vi "Initialize Transfer Group.vi"(5 "FIFO Options":T1, 6 "Transfer Group Status":refnum<class "Transfer Group Status.lvclass">, 7 "id":i32, 8 "error in (no error)":errorcluster, 9 "force inline? (F)":bool, 10 "Transfer Group Buffers":refnum<class "Buffers.lvclass">, 11 "Transfer Group Configuration":T2={"name"="", "direction"=enum."Tx", "cycle timing"={"priority"=0, "decimation"=1, "offset"=0}, "thread"=-1, "settings"=[], "Transfers"=[]} {"Transfers"."channels"."string offset" format="%d bytes"}) -> (0 "error out":errorcluster, 3 "Transfer Group out":refnum<class "Transfer Group.lvclass">)   [LabVIEW 2017, in "DSF Core.lvlib" / "Transfer Group.lvclass"]
uses:
  Transfer Group.lvclass
  Typedefs/DSF Engine Transfer Group Configuration.ctl
  Typedefs/DSF Direction.ctl
  Typedefs/DSF Timing Info.ctl
  Typedefs/DSF Settings Info.ctl
  Typedefs/DSF Engine Transfer Configuration.ctl
  Typedefs/DSF Byte Order.ctl
  Typedefs/DSF Engine Channel Configuration.ctl
  Typedefs/DSF Data Type.ctl
  Buffer/Buffers.lvclass
  Typedefs/DSF FIFO Options.ctl
  Transfer Group Status/Transfer Group Status.lvclass
  Configuration/Required Buffer Size (Transfer).vi
  Transfer/Transfer.lvclass
  DSF Core.lvlib
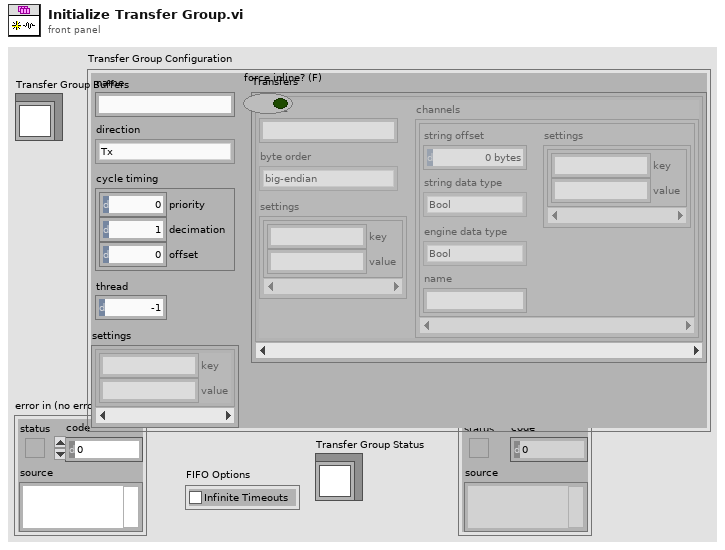
[diagram p1: front panel]
types:
  T1 = typedef "DSF Core.lvlib/DSF FIFO Options.ctl" = cluster{"Infinite Timeouts":bool}
  T2 = typedef "DSF Core.lvlib/DSF Engine Transfer Group Configuration.ctl" = cluster{"name":string, "direction":T3, "cycle timing":T4, "thread":i32, "settings":T5, "Transfers":T6[]}
  T3 = typedef "DSF Core.lvlib/DSF Direction.ctl" = enum8{"Tx", "Rx"}
  T4 = typedef "DSF Core.lvlib/DSF Timing Info.ctl" = cluster{"priority":u64, "decimation":u64, "offset":u64}
  T5 = typedef "DSF Core.lvlib/DSF Settings Info.ctl" = cluster{"key":string, "value":string}[]
  T6 = typedef "DSF Core.lvlib/DSF Engine Transfer Configuration.ctl" = cluster{"name":string, "byte order":T7, "settings":T5, "channels":T8[]}
  T7 = typedef "DSF Core.lvlib/DSF Byte Order.ctl" = enum8{"big-endian", "little-endian"}
  T8 = typedef "DSF Core.lvlib/DSF Engine Channel Configuration.ctl" = cluster{"string offset":u64, "string data type":T9, "engine data type":T9, "name":string, "settings":T5}
  T9 = typedef "DSF Core.lvlib/DSF Data Type.ctl" = enum8{"Bool", "SGL", "DBL", "I8", "I16", "I32", "I64", "U8", "U16", "U32", "U64"}
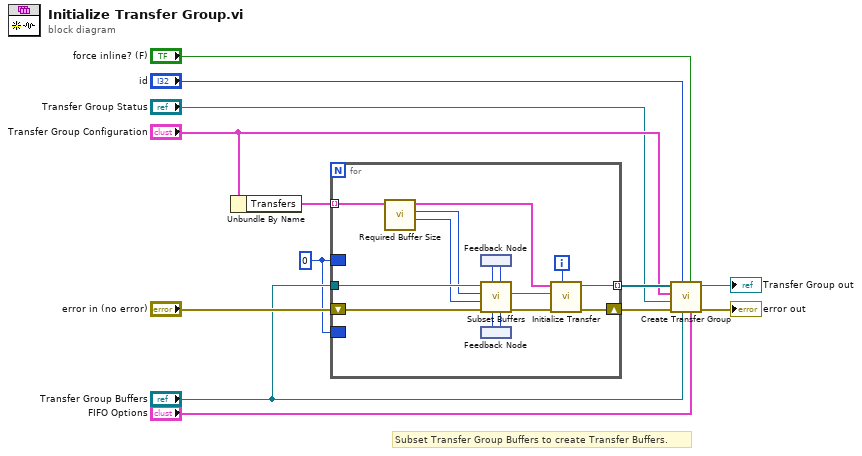
[diagram p0: block diagram]
diagram:
  w6 = u64 0 ("inline buffer size")
  # "Subset Transfer Group Buffers to create Transfer Buffers."
  n1 = Unbundle By Name("Transfer Group Configuration") -> ("Transfers"=w11:T6[])
  n2 = for {
    tunnel: w11 -> [w25] mode=indexing
    tunnel: [w28] -> w9 mode=indexing
    shift-right: [w27] -> w10
    shift-left: "error in (no error)" -> [w23]
    border: w6 -> [_]
    border: w6 -> [_]
    tunnel: "Transfer Group Buffers" -> [w22]
    i -> [w26]
    n3 = call-poly "Required Buffer Size.vi"("Transfer Configuration in"=w25) -> ("total engine buffer size"=w14:u64, "total string buffer size"=w15:u64, "Transfer Configuration out"=w24:T6)  [unwired: 7 in, 1 out]
    n4 = feedback #1() -> (w19:u64)
    n5 = feedback #2() -> (w21:u64)
    n6 = call "Subset Buffers.vi"("inline buffer offset"=w21, "string buffer offset"=w19, "error in (no error)"=w23, "inline buffer size"=w14, "string buffer size"=w15, "Buffers in"=w22) -> ("error out"=w17:errorcluster, "subset Buffers"=w16:refnum<class "Buffers.lvclass">, "inline buffer offset +size"=w20:u64, "string buffer offset + size"=w18:u64)  [unwired: 1 in, 1 out]
    n7 = feedback-in #1(w18) -> ()
    n8 = feedback-in #2(w20) -> ()
    n9 = call "Initialize Transfer.vi"("id"=w26, "error in (no error)"=w17, "Buffers"=w16, "Transfer Configuration"=w24) -> ("error out"=w27:errorcluster, "Transfer out"=w28:refnum<class "Transfer.lvclass">)  [unwired: 6 in]
  }
  n10 = call "Create Transfer Group.vi"("FIFO Options"="FIFO Options", "force inline? (F)"="force inline? (F)", "Buffers"="Transfer Group Buffers", "id"="id", "error in (no error)"=w10, "Transfer Group Status"="Transfer Group Status", "Transfer Group Configuration"="Transfer Group Configuration", "Transfers"=w9) -> ("error out"=→"error out":errorcluster, "Transfer Group out"=→"Transfer Group out":refnum<class "Transfer Group.lvclass">)  [unwired: 2 in]
